vi "Send Message.vi"(4 "waitForResponse":bool=TRUE, 5 "Size":u8, 6 "timeOut (ms)":u32=2000, 7 "Data":u8[](array[numeric]) format="%x", 8 "error in (no error)":errorcluster, 9 "Opcode":u8 format="%x", 10 "Baud Rate":u32=38400, 11 "COM Port":refnum<visa-resource-name>="COM4") -> (0 "error out":errorcluster, 1 "received str":string, 2 "RD Cnt":u32, 3 "Result":bool)   [LabVIEW 2018]
uses:
  RFID GlobalVariable.vi
  <vilib>/Instr/_visa.llb/VISA Configure Serial Port (Instr).vi
panel:
  # "Send Message RFID (rs232)"
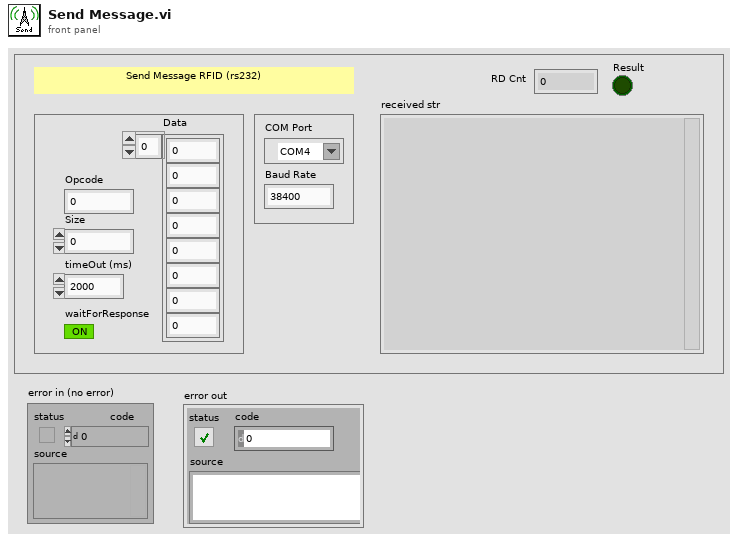
[diagram p1: front panel]
types:
  T1 = enum16{"ALL_GOOD", "ERROR_COMMAND_RESPONSE_TIMEOUT", "ERROR_CORRUPT_RESPONSE", "ERROR_WRONG_OPCODE_RESPONSE", "ERROR_UNKNOWN_OPCODE", "RESPONSE_IS_TEMPERATURE", "RESPONSE_IS_KEEPALIVE", "RESPONSE_IS_TEMPTHROTTLE", "RESPONSE_IS_TAGFOUND", "RESPONSE_IS_NOTAGFOUND", "RESPONSE_IS_UNKNOWN", "RESPONSE_SUCCESS", "RESPONSE_FAIL"}
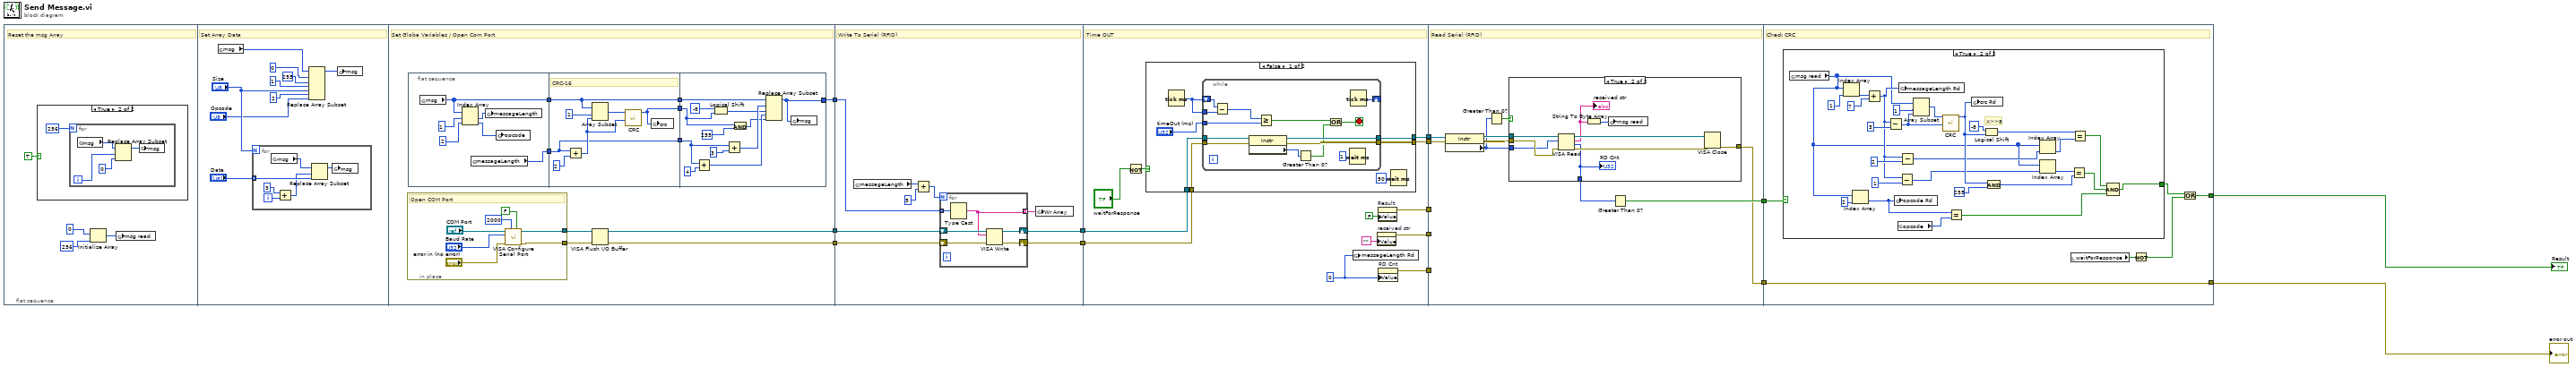
[diagram p0: block diagram]
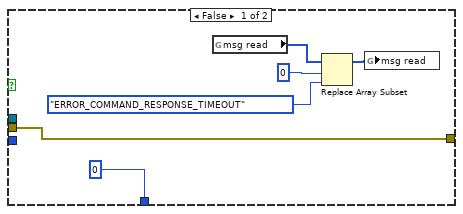
[diagram p4: hidden frame]
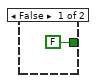
[diagram p5: hidden frame]
diagram:
  n1 = flat-sequence {
    tunnel: [w41] -> w14
    tunnel: [w44] -> w13
    tunnel: [w40] -> w1
    tunnel: w14 -> [w87]
    tunnel: w13 -> [w85]
    tunnel: [w84] -> w12
    tunnel: [w83] -> w11
    tunnel: w1 -> [w86]
    tunnel: w12 -> [w107]
    tunnel: w11 -> [w104]
    tunnel: [w103] -> w10
    tunnel: [w102] -> w9
    tunnel: [w106] -> w8
    tunnel: [w100] -> w5
    tunnel: [w98] -> w2
    tunnel: w10 -> [w139]
    tunnel: w9 -> [w138]
    tunnel: w8 -> [_]
    tunnel: [w132] -> w6
    tunnel: w5 -> [_]
    tunnel: [w131] -> w3
    tunnel: w2 -> [_]
    tunnel: [w160] -> w7
    tunnel: w6 -> [w159]
    tunnel: [w157] -> w4
    tunnel: w3 -> [w160]
    frame #0 {
      # "Reset the msg Array"
      n2 = case shown="True" TRUE {
        frame False {
        }
        frame True {
          n3 = for {
            N: 256 -> [_]
            i -> [w23]
            n4 = global read "RFID GlobalVariable.vi" "msg"() -> (w20:u8[])
            n5 = Replace Array Subset(array=w20, new element=u8 0 ("new element/subarray"), index=w23) -> (w21:u8[])
            n6 = global write "RFID GlobalVariable.vi" "msg"(w21) -> ()
          }
        }
      }
      n7 = Initialize Array(u8 0 ("new element/subarray"), 256) -> (w17:u8[])
      n8 = global write "RFID GlobalVariable.vi" "msg read"(w17) -> ()
    }
    frame #1 {
      # "Set Array Data"
      n9 = global read "RFID GlobalVariable.vi" "msg"() -> (w24:u8[])
      n10 = for {
        N: "Size" -> [_]
        tunnel: "Data" -> [w36] mode=indexing
        i -> [w38]
        n11 = global read "RFID GlobalVariable.vi" "msg"() -> (w33:u8[])
        n12 = Add(x=3, y=w38) -> (x+y=w35:i32)
        n13 = Replace Array Subset(array=w33, new element=w36, index=w35) -> (w34:u8[])
        n14 = global write "RFID GlobalVariable.vi" "msg"(w34) -> ()
      }
      n15 = Replace Array Subset(array=w24, new element #1=u8 255 ("new element/subarray"), index #1=0 ("index"), new element #2="Size", index #2=1 ("index"), new element #3="Opcode", index #3=2 ("index")) -> (w25:u8[])
      n16 = global write "RFID GlobalVariable.vi" "msg"(w25) -> ()
    }
    frame #2 {
      # "Set Globa Variables / Open Com Port"
      n17 = in-place {
        in-place-border: [w52] -> w42
        in-place-border: [w51] -> w39
        # "Open COM Port"
        n18 = call-poly "VISA Configure Serial Port"("VISA resource name"="COM Port", "timeout (10sec)"=u32 2000, "Enable Termination\nChar (T)"=FALSE ("Enable Termination\nChar (T)"), "baud rate (9600)"="Baud Rate", "error in (no error)"="error in (no error)") -> ("VISA resource name out"=w52:refnum<visa-resource-name>, "error out"=w51:errorcluster)  [unwired: 9 in]
      }
      n19 = flat-sequence {
        tunnel: [w59] -> w47
        tunnel: [w58] -> w43
        tunnel: [w62] -> w48
        tunnel: w47 -> [w66]
        tunnel: [w66] -> w46
        tunnel: [w63] -> w45
        tunnel: w43 -> [w63]
        tunnel: w48 -> [w71]
        tunnel: w46 -> [w80]
        tunnel: w45 -> [w70]
        tunnel: [w69] -> w44
        frame #0 {
          n20 = global read "RFID GlobalVariable.vi" "msg"() -> (w59:u8[])
          n21 = Index Array(array=w59, index #1=1 ("index"), index #2=2 ("index")) -> (element #1=w57:u8, element #2=w56:u8)
          n22 = global read "RFID GlobalVariable.vi" "messageLength"() -> (w58:u8)
          n23 = global write "RFID GlobalVariable.vi" "messageLength"(w57) -> ()
          n24 = global write "RFID GlobalVariable.vi" "opcode"(w56) -> ()
        }
        frame #1 {
          # "CRC-16"
          n25 = Add(x=w63, y=u8 2) -> (x+y=w65:u8)
          n26 = Array Subset(array=w66, index=1, length=w65) -> (w68:u8[])
          n27 = call "CRC.vi"("Len"=w65, "u8Buf"=w68) -> ("CRC"=w62:u16)  [unwired: 9 in]
          n28 = global write "RFID GlobalVariable.vi" "crc"(w62) -> ()
        }
        frame #2 {
          n29 = Add(x=w70, y=u8 4) -> (x+y=w76:u8)
          n30 = Logical Shift(y=i8 -8 ("x"), x=w71) -> (x << y=w75:u16)
          n31 = Add(x=w70, y=u8 3) -> (x+y=w78:u8)
          n32 = And(x=w71, y=u8 255) -> (x .and. y?=w74:u16)
          n33 = Replace Array Subset(array=w80, new element #1=w75, index #1=w78, new element #2=w74, index #2=w76) -> (w69:u8[])
          n34 = global write "RFID GlobalVariable.vi" "msg"(w69) -> ()
        }
      }
      n35 = VISA Flush I/O Buffer(VISA resource name=w42, error in (no error)=w39) -> (VISA resource name out=w41:refnum<visa-resource-name>, error out=w40:errorcluster)  [unwired: 1 in]
    }
    frame #3 {
      # "Write To Serial (RFID)"
      n36 = global read "RFID GlobalVariable.vi" "messageLength"() -> (w82:u8)
      n37 = Add(x=w82, y=u8 5) -> (x+y=w88:u8)
      n38 = for {
        N: w88 -> [_]
        shift-right: [w93] -> w84
        shift-left: w87 -> [w95]
        shift-right: [w92] -> w83
        shift-left: w86 -> [w94]
        tunnel: w85 -> [w91] mode=indexing
        tunnel: [w90] -> w81 mode=indexing
        n39 = Type Cast(x=w91) -> (*(type *) &x=w90:string)  [unwired: 1 in]
        n40 = VISA Write(VISA resource name=w95, write buffer=w90, error in (no error)=w94) -> (VISA resource name out=w93:refnum<visa-resource-name>, error out=w92:errorcluster)  [unwired: 1 out]
      }
      n41 = global write "RFID GlobalVariable.vi" "Wr Array"(w81) -> ()
    }
    frame #4 {
      w101 = u32 0 ("RD Cnt")
      # "Time OUT"
      n42 = Not(x="waitForResponse") -> (.not. x?=w97:bool)
      n43 = case shown="False" w97 {
        tunnel: w107 -> [w112 w130]
        tunnel: w104 -> [w111 w129]
        tunnel: [w110 w130] -> w103
        tunnel: [w109 w129] -> w102
        frame False {
          n44 = Tick Count (ms)() -> (millisecond timer value=w113:u32)
          n45 = while {
            tunnel: w112 -> [w122]
            tunnel: w111 -> [w121]
            shift-right: [w127] -> _
            shift-left: w113 -> [w125]
            tunnel: "timeOut (ms)" -> [w126]
            tunnel: w113 -> [w124]
            tunnel: [w120] -> w110
            tunnel: [w119] -> w109
            stop <- w117 stop-if-true
            n46 = Subtract(x=w125, y=w124) -> (x-y=w123:u32)
            n47 = property class="Instr"(reference=w122, error in=w121) -> (reference out=w120:refnum<visa-resource-name>, error out=w119:errorcluster, "Serial Settings:Number of Bytes at Serial Port"=w118:u32)
            n48 = Greater Or Equal?(x=w123, y=w126) -> (x >= y?=w116:bool)
            n49 = Greater Than 0?(x=w118) -> (x > 0?=w115:bool)
            n50 = Or(x=w116, y=w115) -> (x .or. y?=w117:bool)
            n51 = Wait (ms)(milliseconds to wait=u32 1) -> ()  [unwired: 1 out]
            n52 = Tick Count (ms)() -> (millisecond timer value=w127:u32)
          }
          n53 = Wait (ms)(milliseconds to wait=u32 50) -> ()  [unwired: 1 out]
        }
        frame True {
        }
      }
      n54 = global write "RFID GlobalVariable.vi" "messageLength Rd"(w101) -> ()
      n55 = property on="received str" class="Str"("Value"="") -> (error out=w106:errorcluster)  [unwired: 2 in, 1 out]
      n56 = property on="Result" class="Bool (strict)"("Value"=FALSE ("CRC Rd")) -> (error out=w100:errorcluster)  [unwired: 2 in, 1 out]
      n57 = property on="RD Cnt" class="DigNum (strict)"("Value"=w101) -> (error out=w98:errorcluster)  [unwired: 2 in, 1 out]
    }
    frame #5 {
      # "Read Serial (RFID)"
      n58 = property class="Instr"(reference=w139, error in=w138) -> (reference out=w137:refnum<visa-resource-name>, error out=w136:errorcluster, "Serial Settings:Number of Bytes at Serial Port"=w135:u32)
      n59 = Greater Than 0?(x=w135) -> (x > 0?=w134:bool)
      n60 = case shown="True" w134 {
        tunnel: [w145 w154] -> w131
        tunnel: w137 -> [_ w153]
        tunnel: w136 -> [w145 w152]
        tunnel: w135 -> [_ w147]
        tunnel: [0 w146] -> w133
        frame False {
          n61 = global read "RFID GlobalVariable.vi" "msg read"() -> (w144:u8[])
          n62 = Replace Array Subset(array=w144, new element=T1."ERROR_COMMAND_RESPONSE_TIMEOUT" ("Return"), index=0) -> (w143:u8[])
          n63 = global write "RFID GlobalVariable.vi" "msg read"(w143) -> ()
        }
        frame True {
          n64 = VISA Read(VISA resource name=w153, byte count=w147, error in (no error)=w152) -> (VISA resource name out=w151:refnum<visa-resource-name>, read buffer=w149:string, return count=w146:u32, error out=w150:errorcluster)
          "received str" <- w149
          "RD Cnt" <- w146
          n65 = String To Byte Array(string=w149) -> (unsigned byte array=w148:u8[])
          n66 = global write "RFID GlobalVariable.vi" "msg read"(w148) -> ()
          n67 = VISA Close(VISA resource name=w151, error in (no error)=w150) -> (error out=w154:errorcluster)
        }
      }
      n68 = Greater Than 0?(x=w133) -> (x > 0?=w132:bool)
    }
    frame #6 {
      # "Check CRC"
      n69 = case shown="True" w159 {
        tunnel: [FALSE w162] -> w158
        frame False {
        }
        frame True {
          # "X>>8"
          n70 = global read "RFID GlobalVariable.vi" "msg read"() -> (w169:u8[])
          n71 = Index Array(array=w169, index=1) -> (element=w187:u8)
          n72 = Index Array(array=w169, index=2) -> (element=w167:u8)
          n73 = Add(x=w187, y=u8 7) -> (x+y=w178:u8)
          n74 = Subtract(x=w178, y=u8 3) -> (x-y=w182:u8)
          n75 = global write "RFID GlobalVariable.vi" "opcode Rd"(w167) -> ()
          n76 = global read "RFID GlobalVariable.vi" "opcode"() -> (w166:u8)
          n77 = global write "RFID GlobalVariable.vi" "messageLength Rd"(w178) -> ()
          n78 = Subtract(x=w178, y=u8 1) -> (x-y=w175:u8)
          n79 = Subtract(x=w178, y=u8 2) -> (x-y=w176:u8)
          n80 = Array Subset(array=w169, index=1, length=w182) -> (w185:u8[])
          n81 = call "CRC.vi"("Len"=w182, "u8Buf"=w185) -> ("CRC"=w180:u16)  [unwired: 9 in]
          n82 = Equal?(x=w167, y=w166) -> (x = y?=w163:bool)
          n83 = global write "RFID GlobalVariable.vi" "crc Rd"(w180) -> ()
          n84 = Logical Shift(y=i8 -8 ("x"), x=w180) -> (x << y=w174:u16)
          n85 = And(x=w180, y=u8 255) -> (x .and. y?=w171:u16)
          n86 = Index Array(array=w169, index=w176) -> (element=w173:u8)
          n87 = Index Array(array=w169, index=w175) -> (element=w172:u8)
          n88 = Equal?(x=w172, y=w171) -> (x = y?=w164:bool)
          n89 = Equal?(x=w174, y=w173) -> (x = y?=w165:bool)
          n90 = Compound Arithmetic op=AND(w165, w164, w163) -> (w162:bool)
        }
      }
      n91 = local read "waitForResponse"() -> (w156:bool)
      n92 = Not(x=w156) -> (.not. x?=w155:bool)
      n93 = Or(x=w158, y=w155) -> (x .or. y?=w157:bool)
    }
  }
  "error out" <- w7
  "Result" <- w4
